vi "Microchip 93C86 Write.vi"() -> ()   [LabVIEW 2015]
doc: "This example shows a more generalized way to use the SPI advanced API to write data. It allows the user to change the following parameters: page size, write delay, the endianness of the address bytes, and the number of bytes in an address.\n\nThe parameters will have the following effects:\n\nTarget Page Size (bytes): This places an additional constraint on the amount of bytes written. The smaller value will be used, and that number of bytes written.\nWrite Delay Between Pages (ms): This will force a mandatory delay after writing bytes to a device.\nData Address Width: This will allow the user to specify the EEPROM Data Address as either 1 or 2 bytes.\nData Address Endianness: This control will change the ordering of the bytes in the EEPROM Data Address, note that this only has an effect if there are 2 bytes in the address.\n\nFor connection information see the NI-845x Hardware and Software manual and the manual for your specific SPI device."
uses:
  <vilib>/ni845x/ni845x.llb/ni845xControl.ctl
  <vilib>/ni845x/ni845x.llb/NI-845x SPI Script Ms Delay.vi
  <vilib>/ni845x/ni845x.llb/NI-845x SPI Close Script Reference.vi
  <resource>/objmgr/NI845x.rc
panel:
  in  "Bit Pattern":T1(ring)
  in  "I/O Voltage Level":i32(ring)=33 items=["3.3V"=33, "2.5V"=25, "1.8V"=18, "1.5V"=15, "1.2V"=12]
  in  "Chip Select":u32
  in  "Data Address Width":enum16{"1 Byte", "2 Byte"}(ring)=enum."2 Byte"
  in  "Data Address Endianness":bool=TRUE
  in  "Write Delay Between Pages (ms)":u32=3
  in  "Target Page Size (bytes)":u32=2
  in  "Device":T2="NI-8451"
  in  "EEPROM Data Address":u8 format="%.0x"
  in  "Number of Bytes to Write":u32=16384
  in  "Clock Rate (kHz)":u16=2000
  out "Data Bytes Written":u8[](array[numeric]) format="%x"
  # "See VI Info <Ctrl+I> for more information on how to use this example"
  # "Device Configuration"
  # "SPI Data"
  # "SPI Slave Configuration"
  # "Big Endian"
  # "Note 1: Microchip 93C76/86\nEEPROM devices DC signal levels\nare 2.0V (min) to Vcc (5.0V) +1V\nmax.\n\nNote 2: NI-8451 max signal\nlevel is 3.5V so recommended\nI/O voltage of 3.3V is OK."
  # "Little Endian"
  # "Note: WRITE cycle takes 3 ms per word (typical)"
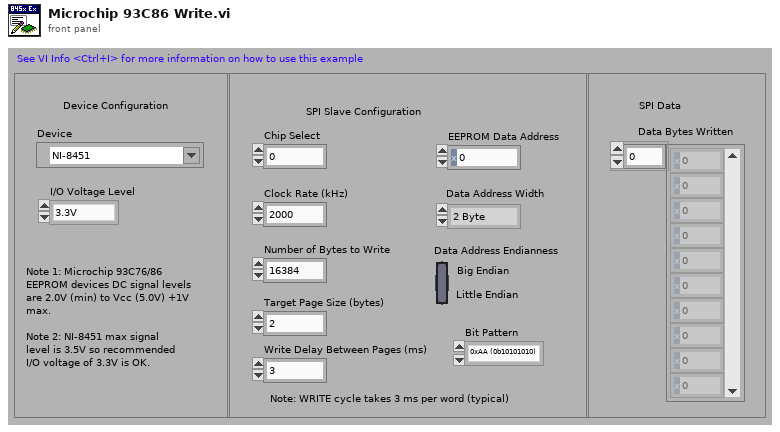
[diagram p1: front panel]
types:
  T1 = enum16{"0xAA (0b10101010)", "0x55 (0b01010101)", "All ONES", "All ZEROES"}
  T2 = typedef "ni845xControl.ctl" = refnum<k21>
  T3 = typedef "ni845xSpiScriptControl.ctl" = refnum<k20>
  T4 = cluster{"EEPROM Address":u16, "Length":u32, "Data Index":u32}[]
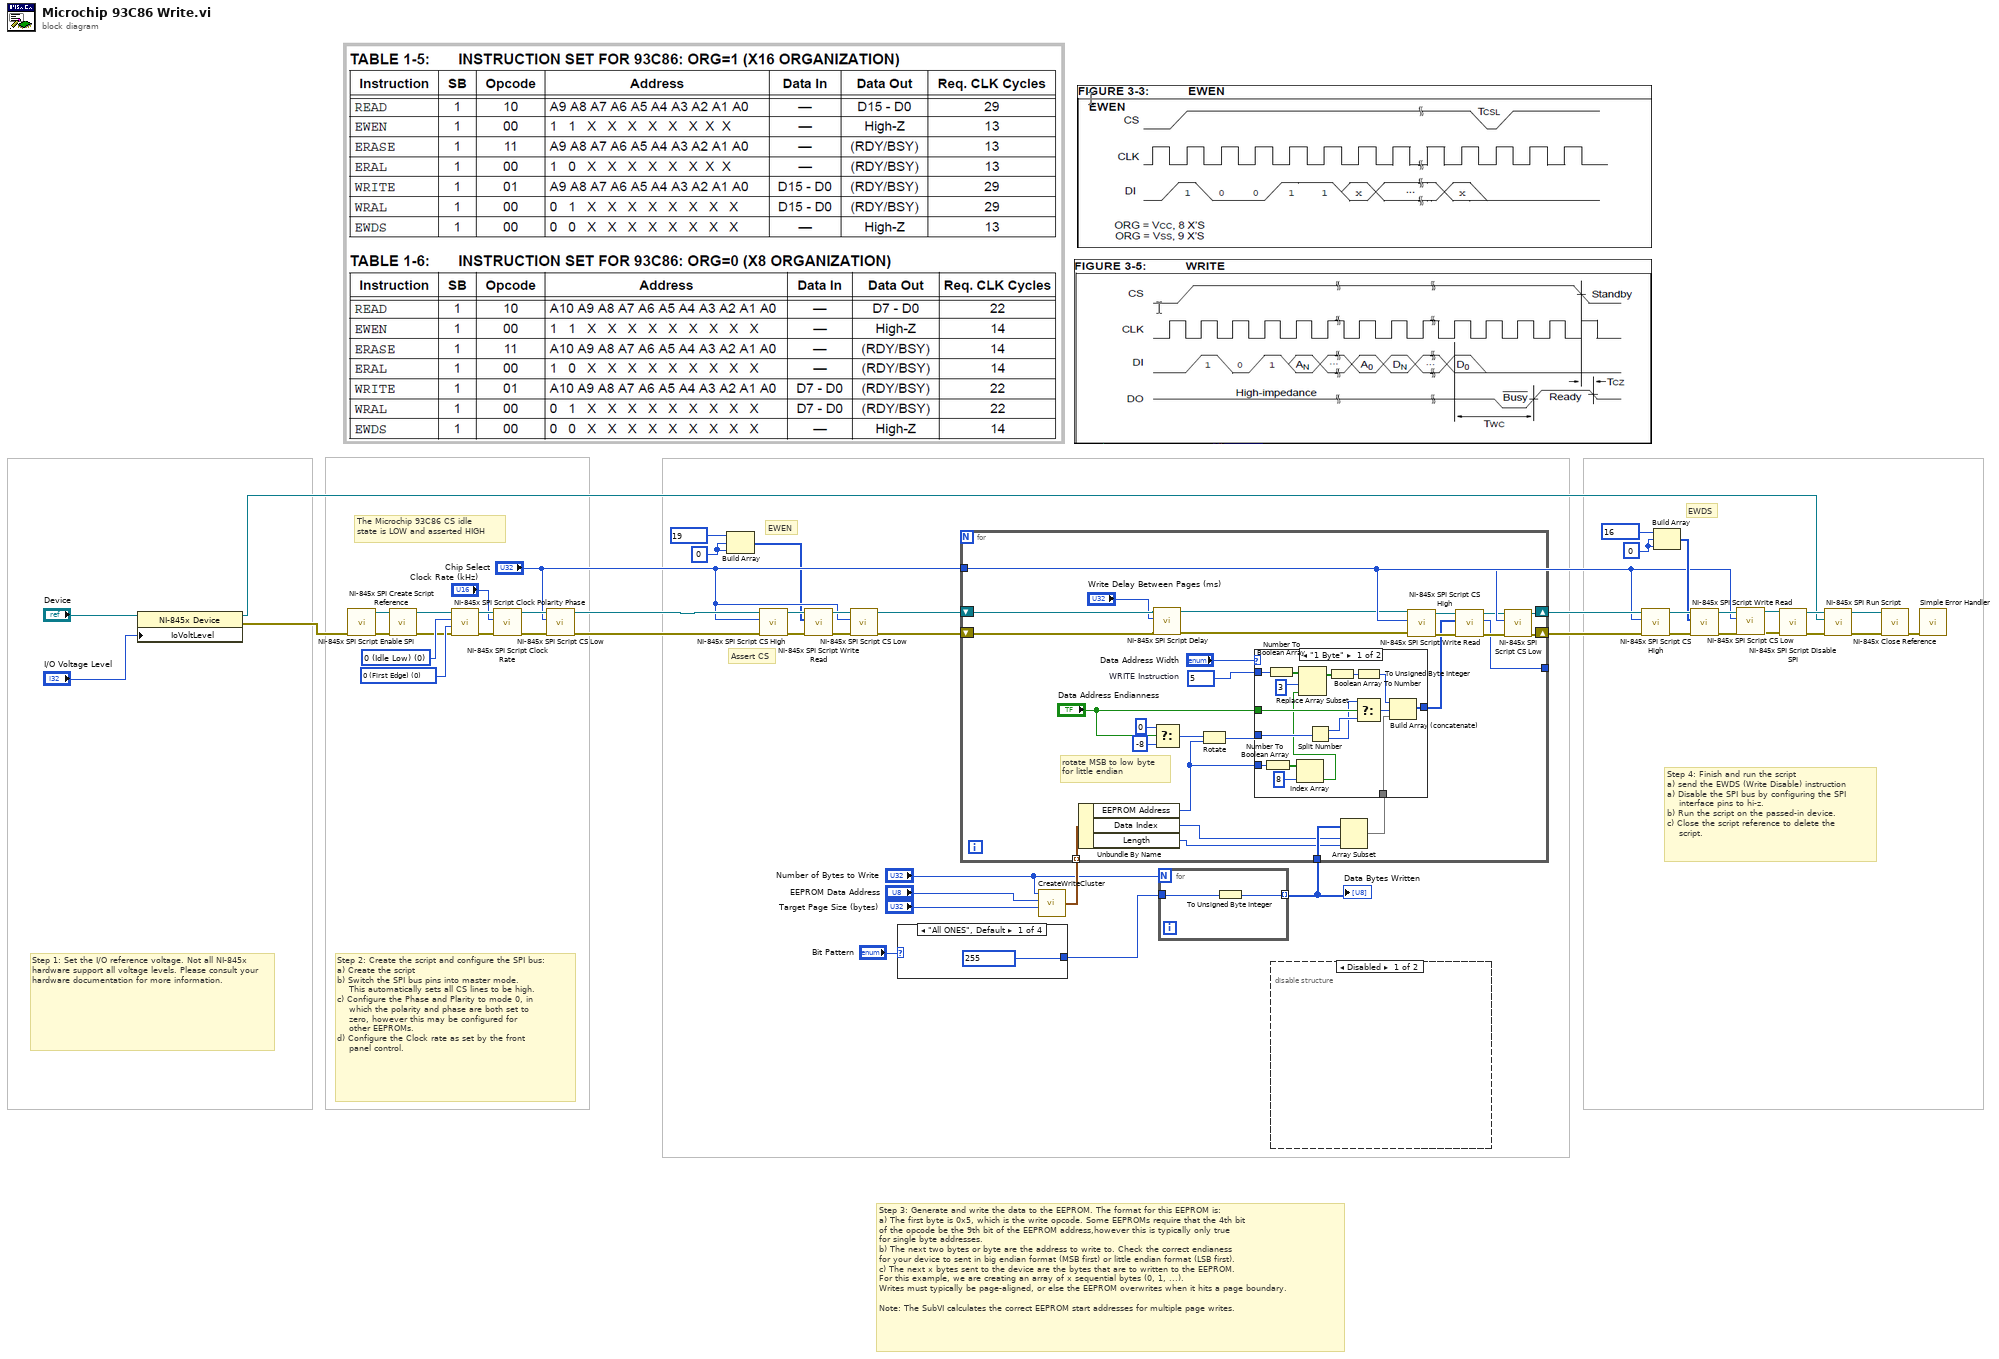
[diagram p0: block diagram]
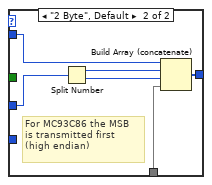
[diagram p3: hidden frame]
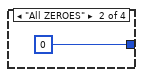
[diagram p4: hidden frame]
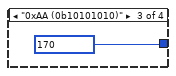
[diagram p5: hidden frame]
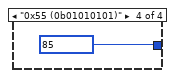
[diagram p6: hidden frame]
diagram:
  w5 = u8 0
  w4 = u8 0
  w39 = 0 items=["0 (First Edge)", "1 (Second Edge)"] ("clock phase (0)")
  w40 = 0 items=["0 (Idle Low)", "1 (Idle High)"] ("clock polarity (0)")
  # "Assert CS"
  # "EWEN"
  # "The Microchip 93C86 CS idle\nstate is LOW and asserted HIGH"
  # "EWDS"
  # "Step 1: Set the I/O reference voltage. Not all NI-845x hardware support all voltage levels. Please consult your hardware documentation for more information."
  # "Step 4: Finish and run the script\na) send the EWDS (Write Disable) instruction\na) Disable the SPI bus by configuring the SPI \n    interface pins to hi-z.\nb) Run the script on the passed-in device. \nc) Close the script reference to delete the \n    script."
  # "Step 3: Generate and write the data to the EEPROM. The format for this EEPROM is:\na) The first byte is 0x5, which is the write opcode. Some EEPROMs require that the 4th bit \nof the opcode be the 9th bit of the EEPROM address,however this is typically only true \nfor single byte addresses.\nb) The next two bytes or byte are the address to write to. Check the correct endianess \nfor your device to sent in big endian format (MSB first) or little endian format (LSB first).\nc) The next x bytes sent to the device are the bytes that are to written to the EEPROM. \nFor this example, we are creating an array of x sequential bytes (0, 1, ...). \nWrites must typically be page-aligned, or else the EEPROM overwrites when it hits a page boundary.\n\nNote: The SubVI calculates the correct EEPROM start addresses for multiple page writes."
  # "Step 2: Create the script and configure the SPI bus:\na) Create the script\nb) Switch the SPI bus pins into master mode. \n    This automatically sets all CS lines to be high.\nc) Configure the Phase and Plarity to mode 0, in \n    which the polarity and phase are both set to \n    zero, however this may be configured for \n    other EEPROMs. \nd) Configure the Clock rate as set by the front \n    panel control."
  n1 = property on="Property Node" class="NI-845x Device"(reference="Device", "IoVoltLevel"="I/O Voltage Level") -> (reference out=w31:T2, error out=w28:errorcluster)  [unwired: 1 in]
  n2 = call <vilib>:"NI-845x SPI Create Script Reference.vi"("error in (no error)"=w28) -> ("error out"=w37:errorcluster, "spi script reference"=w38:T3)  [unwired: 9 out]
  n3 = call <vilib>:"NI-845x SPI Script Enable SPI.vi"("error in (no error)"=w37, "spi script reference in"=w38) -> ("error out"=w21:errorcluster, "spi script reference out"=w20:T3)  [unwired: 8 out]
  n4 = call <vilib>:"NI-845x SPI Script Clock Polarity Phase.vi"("error in (no error)"=w21, "clock phase (0)"=w39, "clock polarity (0)"=w40, "spi script reference in"=w20) -> ("error out"=w44:errorcluster, "spi script reference out"=w43:T3)  [unwired: 2 in, 4 out]
  n5 = call <vilib>:"NI-845x SPI Script Clock Rate.vi"("error in (no error)"=w44, "clock rate in kHz (1000)"="Clock Rate (kHz)", "spi script reference in"=w43) -> ("error out"=w17:errorcluster, "spi script reference out"=w16:T3)  [unwired: 1 in, 6 out]
  n6 = call <vilib>:"NI-845x SPI Script CS Low.vi"("error in (no error)"=w17, "chip select (0)"="Chip Select", "spi script reference in"=w16) -> ("spi script reference out"=w15:T3)  [unwired: 7 in, 1 out]
  n7 = Build Array(u8 19, w5, w5) -> (w6:u8[])
  n8 = call <vilib>:"NI-845x SPI Script CS High.vi"("error in (no error)"=w17, "chip select (0)"="Chip Select", "spi script reference in"=w15) -> ("error out"=w10:errorcluster, "spi script reference out"=w9:T3)  [unwired: 7 in]
  n9 = call <vilib>:"NI-845x SPI Script Write Read.vi"("error in (no error)"=w10, "write data"=w6, "spi script reference in"=w9) -> ("error out"=w8:errorcluster, "spi script reference out"=w7:T3)  [unwired: 1 in, 6 out]
  n10 = call <vilib>:"NI-845x SPI Script CS Low.vi"("error in (no error)"=w8, "chip select (0)"="Chip Select", "spi script reference in"=w7) -> ()  [unwired: 7 in, 2 out]
  n11 = case shown="\"All ONES\", Default" "Bit Pattern" {
    tunnel: [255 0 170 85] -> w12
    frame "All ONES", Default {
    }
    frame "All ZEROES" {
    }
    frame "0xAA (0b10101010)" {
    }
    frame "0x55 (0b01010101)" {
    }
  }
  n12 = call "CreateWriteCluster.vi"("Page Size in Bytes"="Target Page Size (bytes)", "EEPROM Starting Address"="EEPROM Data Address", "Number of Bytes to Write"="Number of Bytes to Write") -> ("Array of Write Cluster Information"=w33:T4)  [unwired: 1 in]
  n13 = for {
    N: "Number of Bytes to Write" -> [_]
    tunnel: [w51] -> w3 mode=indexing
    tunnel: w12 -> [w50]
    n14 = To Unsigned Byte Integer(number=w50) -> (unsigned 8bit integer=w51:u8)
  }
  "Data Bytes Written" <- w3
  n15 = for {
    tunnel: w33 -> [w78] mode=indexing
    tunnel: w3 -> [w77]
    tunnel: "Chip Select" -> [w72]
    shift-right: [w76] -> w27
    shift-left: w17 -> [w74]
    shift-right: [w75] -> w26
    shift-left: w15 -> [w73]
    tunnel: [w59] -> _
    w56 = u8 5  # WRITE Instruction
    # "rotate MSB to low byte\nfor little endian"
    n16 = Unbundle By Name(w78) -> ("EEPROM Address"=w53:u16, "Data Index"=w65:u32, "Length"=w64:u32)
    n17 = call-poly <vilib>:"NI-845x SPI Script Delay.vi"("error in (no error)"=w74, "delay in milliseconds (0)"="Write Delay Between Pages (ms)", "spi script reference in"=w73) -> ("error out"=w61:errorcluster, "spi script reference out"=w60:T3)  [unwired: 7 out]
    n18 = Select(t=i16 0, s="Data Address Endianness", f=i16 -8) -> (s? t:f=w66:i16)
    n19 = Rotate(1:w53, 2:w66) -> (0:w54:u16)
    n20 = Array Subset(array=w77, index=w65, length=w64) -> (w52:u8[])
    n21 = case shown="\"1 Byte\"" "Data Address Width" {
      tunnel: [w95 w101] -> w58
      tunnel: w54 -> [w94 w97]
      tunnel: w56 -> [w84 w98]
      tunnel: "Data Address Endianness" -> [w92 _]
      tunnel: w52 -> [w83 w96]
      tunnel: w53 -> [w80 _]
      frame "1 Byte" {
        n22 = Number To Boolean Array(number=w80) -> (Boolean array=w82:bool[])
        n23 = Number To Boolean Array(number=w84) -> (Boolean array=w89:bool[])
        n24 = Index Array(array=w82, index=8) -> (element=w79:bool)
        n25 = Replace Array Subset(array=w89, new element=w79, index=3) -> (w87:bool[])
        n26 = Split Number(x=w94) -> (hi(x)=w93:u8, lo(x)=w91:u8)
        n27 = Boolean Array To Number(Boolean array=w87) -> (number=w86:u32)
        n28 = To Unsigned Byte Integer(number=w86) -> (unsigned 8bit integer=w85:u8)
        n29 = Select(t=w91, s=w92, f=w93) -> (s? t:f=w90:u8)
        n30 = Build Array (concatenate)(w85, w90, w83) -> (w95:u8[])
      }
      frame "2 Byte", Default {
        # "For MC93C86 the MSB\nis transmitted first\n(high endian)"
        n31 = Split Number(x=w97) -> (hi(x)=w99:u8, lo(x)=w100:u8)
        n32 = Build Array (concatenate)(w98, w99, w100, w96) -> (w101:u8[])
      }
    }
    n33 = call <vilib>:"NI-845x SPI Script CS High.vi"("error in (no error)"=w61, "chip select (0)"=w72, "spi script reference in"=w60) -> ("error out"=w62:errorcluster, "spi script reference out"=w63:T3)  [unwired: 7 in]
    n34 = call <vilib>:"NI-845x SPI Script Write Read.vi"("error in (no error)"=w62, "write data"=w58, "spi script reference in"=w63) -> ("error out"=w70:errorcluster, "script read index"=w59:u32, "spi script reference out"=w69:T3)  [unwired: 1 in, 5 out]
    n35 = call <vilib>:"NI-845x SPI Script CS Low.vi"("error in (no error)"=w70, "chip select (0)"=w72, "spi script reference in"=w69) -> ("error out"=w76:errorcluster, "spi script reference out"=w75:T3)  [unwired: 7 in]
  }
  n36 = disable-structure shown="Disabled" {
    frame Disabled {
    }
    frame Enabled {
    }
  }
  n37 = call <vilib>:"NI-845x SPI Script CS High.vi"("error in (no error)"=w27, "chip select (0)"="Chip Select", "spi script reference in"=w26) -> ()  [unwired: 7 in, 2 out]
  n38 = Build Array(u8 16, w4, w4) -> (w18:u8[])
  n39 = call <vilib>:"NI-845x SPI Script Write Read.vi"("error in (no error)"=w27, "write data"=w18, "spi script reference in"=w26) -> ("error out"=w25:errorcluster, "spi script reference out"=w24:T3)  [unwired: 1 in, 6 out]
  n40 = call <vilib>:"NI-845x SPI Script CS Low.vi"("error in (no error)"=w25, "chip select (0)"="Chip Select", "spi script reference in"=w24) -> ("error out"=w23:errorcluster, "spi script reference out"=w22:T3)  [unwired: 7 in]
  n41 = call <vilib>:"NI-845x SPI Script Disable SPI.vi"("error in (no error)"=w23, "spi script reference in"=w22) -> ("error out"=w45:errorcluster, "spi script reference out"=w42:T3)  [unwired: 8 out]
  n42 = call <vilib>:"NI-845x SPI Run Script.vi"("error in (no error)"=w45, "device reference in"=w31, "spi script reference in"=w42) -> ("error out"=w1:errorcluster, "spi script reference out"=w2:T3)  [unwired: 1 in, 6 out]
  n43 = call-poly <vilib>:"NI-845x Close Reference.vi"("error in (no error)"=w1, "spi script reference"=w2) -> ("error out"=w36:errorcluster)  [unwired: 9 out]
  n44 = call <vilib>:"Simple Error Handler.vi"("error in (no error)"=w36) -> ()  [unwired: 1 in, 8 out]
